vi "Import Options Dialog.vi"(8 "error in (no error)":errorcluster) -> (0 "error out":errorcluster, 1 "Overwrite Existing Channels?":bool, 2 "Overwrite Device Settings?":bool)   [LabVIEW 2020, in "Modbus Master System Explorer.lvlib"]
uses:
  Modbus Master System Explorer.lvlib
panel:
  in  "Stop":bool
  in  "Overwrite Existing Channels":bool
  in  "Overwrite Device Settings":bool
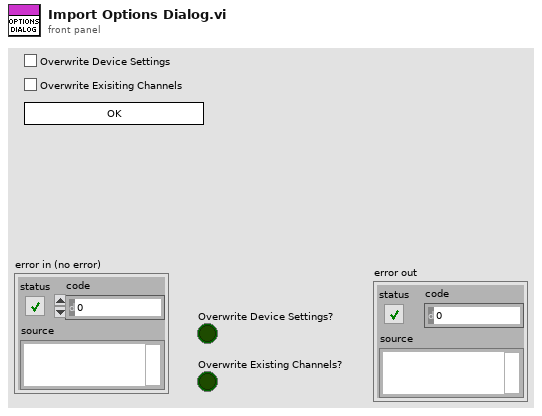
[diagram p1: front panel]
types:
  T1 = enum32{"Invalid", "Standard", "Closed", "Hidden", "Minimized", "Maximized"}
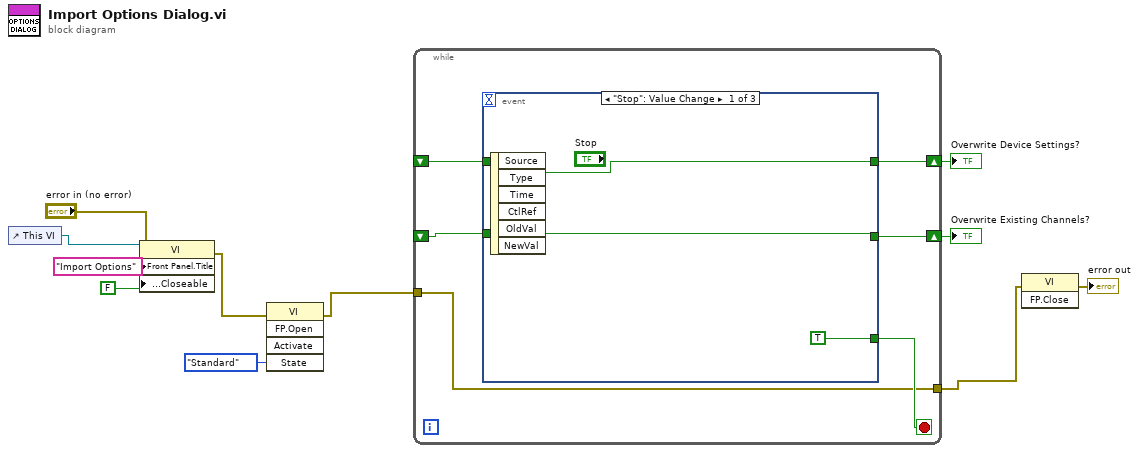
[diagram p0: block diagram]
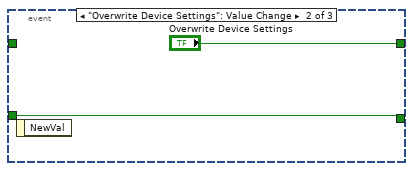
[diagram p2: hidden frame]
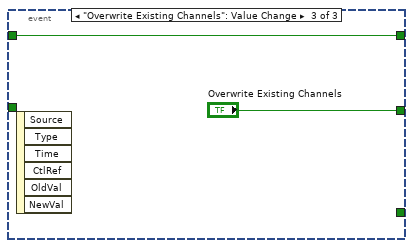
[diagram p3: hidden frame]
diagram:
  n1 = control-ref of="This VI"() -> (w7:refnum<vi>)
  n2 = property class="VI"(reference=w7, error in="error in (no error)", "Front Panel.Title"="Import Options" ("Front Panel Window:Title"), "Front Panel.Closeable"=FALSE ("Front Panel Window:Closeable")) -> (error out=w5:errorcluster)  [unwired: 1 out]
  n3 = invoke class="VI" method="FP.Open"(error in=w5, "State"=T1."Standard") -> (error out=w4:errorcluster)  [unwired: 3 in, 4 out]
  n4 = while {
    shift-right: [w16] -> w11
    shift-left: _ -> [w13]
    shift-right: [w15] -> w10
    shift-left: _ -> [w14]
    tunnel: w4 -> [w12]
    tunnel: [w12] -> w3
    stop <- w17 stop-if-true
    n5 = event shown="[0] \"Stop\": Value Change" {
      selector: _ -> [_ _ _]
      dyn-events: _ -> [_ _ _]
      timeout: _ -> [_ _ _]
      tunnel: [TRUE _ _] -> w17
      tunnel: [w19 "Overwrite Device Settings" w23] -> w16
      tunnel: [w18 w21 "Overwrite Existing Channels"] -> w15
      tunnel: w14 -> [w18 w21 _]
      tunnel: w13 -> [w19 _ w23]
      event "Stop": Value Change {
        n6 = event-data() -> ()  [unwired: 1 in, 6 out]
      }
      event "Overwrite Device Settings": Value Change {
        n7 = event-data() -> ()  [unwired: 1 in, 1 out]
      }
      event "Overwrite Existing Channels": Value Change {
        n8 = event-data() -> ()  [unwired: 1 in, 6 out]
      }
    }
  }
  "Overwrite Device Settings?" <- w11
  "Overwrite Existing Channels?" <- w10
  n9 = invoke class="VI" method="FP.Close"(error in=w3) -> (error out=→"error out":errorcluster)  [unwired: 2 in, 2 out]
